vi "Reset Global Variable.vi"(8 "error in (no error)":errorcluster) -> (0 "error out":errorcluster)   [LabVIEW 2020, in "Global Fixture Test Double.lvclass"]
uses:
  Global Fixture Test Double.lvclass
  Global Variable.vi
  Global Fixture Test Double.lvclass/Global Fixture Test Double.ctl
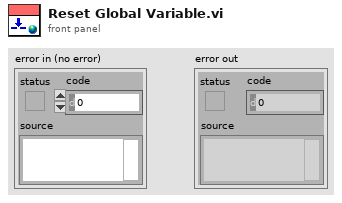
[diagram p1: front panel]
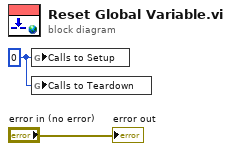
[diagram p0: block diagram]
diagram:
  w1 = 0 ("Calls to Setup")
  n1 = global write "Global Variable.vi" "Calls to Setup"(w1) -> ()
  n2 = global write "Global Variable.vi" "Calls to Teardown"(w1) -> ()
  "error out" <- "error in (no error)"
